vi "Fluke 190 Series II Acquire Waveform.vi"() -> ()   [LabVIEW 2014]
doc: "This example shows how to read a waveform on specific trace number and channel from the instrument."
uses:
  Fluke 190 Series II.lvlib
panel:
  out "Waveform":cluster{dbl[], "Max Data":dbl[]}[](graph)
  out "X Unit":string
  out "Y Unit":string
  in  "Channel (1: Channel A)":i32(ring)=1 items=["Channel A"=1, "Channel B"=2, "Channel C"=5, "Channel D"=6]
  in  "Trace Number (0: Scope Trace or Record)":i32(ring) items=["Scope Trace or Record", "Trend Plot", "Persistence", "Reference Trace", "Spectrum"]
  in  "VISA resource name":refnum<visa-resource-name>
  # "(c) 2013-2014 National Instruments.  ALL RIGHTS RESERVED."
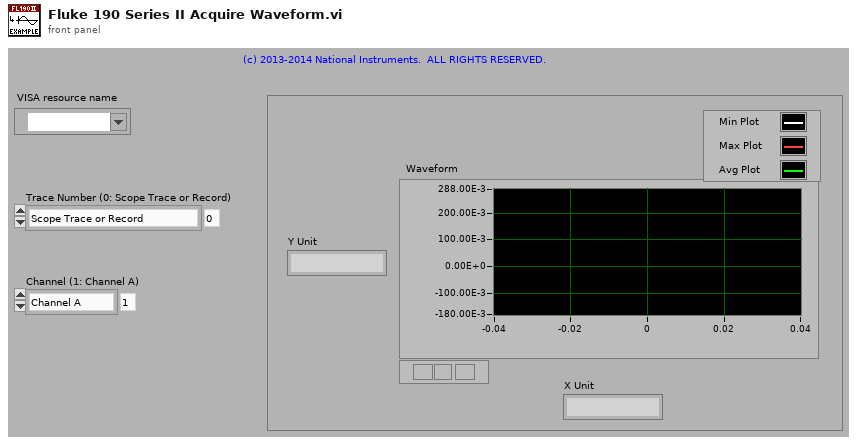
[diagram p1: front panel]
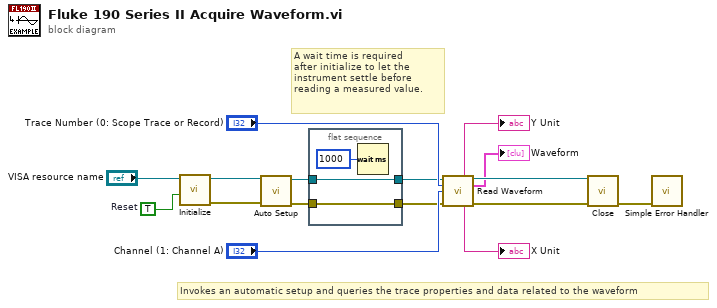
[diagram p0: block diagram]
diagram:
  w16 = TRUE  # Reset
  # "A wait time is required\nafter initialize to let the\ninstrument settle before\nreading a measured value."
  # "Invokes an automatic setup and queries the trace properties and data related to the waveform"
  n1 = call "Initialize.vi"("Reset (True)"=w16, "VISA resource name"="VISA resource name") -> ("error out"=w1:errorcluster, "VISA resource name out"=w2:refnum<visa-resource-name>)  [unwired: 2 in, 6 out]
  n2 = call "Auto Setup.vi"("error in (no error)"=w1, "VISA resource name"=w2) -> ("error out"=w4:errorcluster, "VISA resource name out"=w6:refnum<visa-resource-name>)  [unwired: 8 out]
  n3 = flat-sequence {
    tunnel: w6 -> [w18]
    tunnel: [w18] -> w5
    tunnel: w4 -> [w17]
    tunnel: [w17] -> w3
    frame #0 {
      n4 = Wait (ms)(milliseconds to wait=u32 1000) -> ()  [unwired: 1 out]
    }
  }
  n5 = call "Read Waveform.vi"("VISA resource name"=w5, "Trace Number (0: Scope Trace or Record)"="Trace Number (0: Scope Trace or Record)", "Channel (1: Channel A)"="Channel (1: Channel A)", "error in (no error)"=w3) -> ("Y Unit"=→"Y Unit":string, "VISA resource name out"=w12:refnum<visa-resource-name>, "Waveform"=→"Waveform":cluster{dbl[], "Max Data":dbl[]}[], "X Unit"=→"X Unit":string, "error out"=w11:errorcluster)  [unwired: 7 out]
  n6 = call "Close.vi"("error in (no error)"=w11, "VISA resource name"=w12) -> ("error out"=w10:errorcluster)  [unwired: 9 out]
  n7 = call <vilib>:"Simple Error Handler.vi"("error in (no error)"=w10) -> ()  [unwired: 1 in, 8 out]
